vi "Rectangular Target Processing.vi"() -> ()   [LabVIEW 2011]
doc: "This VI demonstrates how to do target processing on a laptop computer. It uses the same MJPG VI as the dashboard, sets a few of the important camera properties that impact processing, and carries out the same processing steps as the RT example also included in this project."
uses:
  <vilib>/Rock Robotics/WPI/Camera/WPI_CameraImageSize.ctl
  <vilib>/Rock Robotics/WPI/Camera/WPI_CameraWhite Balance Values.ctl
  <vilib>/vision/NI_Vision_Development_Module.lvlib
panel:
  in  "Camera Settings":T2={"FPS"=30, "Compression"=30, "Image Size"=enum."320x240"}
  in  "Camera IP Address":string="192.168.0.90"
  in  "Camera Type":enum16{"206", "1011"}(ring)
  out "Target Info":T3(array[cluster])
  in  "Area Size Limit":i32=444
  in  "Particle Count Limit":i32=10
  in  "Score Limits":T4={"Rect Coverage"=76.0, "Aspect Ratio"=70.0, "X Edge Strength"=40.0, "Y Edge Strength"=60.0}
  in  "Processing":enum32{"Color", "Intensity", "Intensity Open"}(tab)
  in  "Luminance":i32=255
  in  "Saturation":i32=255
  in  "Hue":i32(knob)=65 scale=0.0..255.0
  in  "Margins":cluster{"Hue":i32, "Sat":i32, "Lum":i32}={"Hue"=9, "Sat"=40, "Lum"=19} {"Sat" scale=0.0..40.0; "Lum" scale=0.0..40.0; "Hue" scale=0.0..40.0}
  in  "Range":cluster{"Lower value":sgl, "Upper value":sgl}={"Lower value"=150.0, "Upper value"=255.0} {"Lower value" scale=0.0..255.0; "Upper value" scale=0.0..255.0}
  in  "Range":cluster{"Lower value":sgl, "Upper value":sgl}={"Lower value"=150.0, "Upper value"=255.0} {"Lower value" scale=0.0..255.0; "Upper value" scale=0.0..255.0}
  in  "Annotate":bool=TRUE
  out "Processed Image":T5(plugin-control)
  out "Original Image":T5(plugin-control)
  # "Information:\nProcessing can be based on color or light intensity.\nParticles within the image are scored by rectangle coverage, aspect ratio, and\nfor being hollow with a bold edge. A particle is considered a target if all scores\nare above the score limits you set. Particles can be annotated -- surrounded by\na rectangle and scores drawn to the left .\nTo control the number of particles being scored, use the count limit and the size\nlimit.\nBe sure to set the Camera IP before running. The distance uses the camera type\nto index lens view angle."
  # "Click in the image to select target the color for processing."
  # "Green scores are above the limit, orange are below. Inner/outer rect\nindicates all passed."
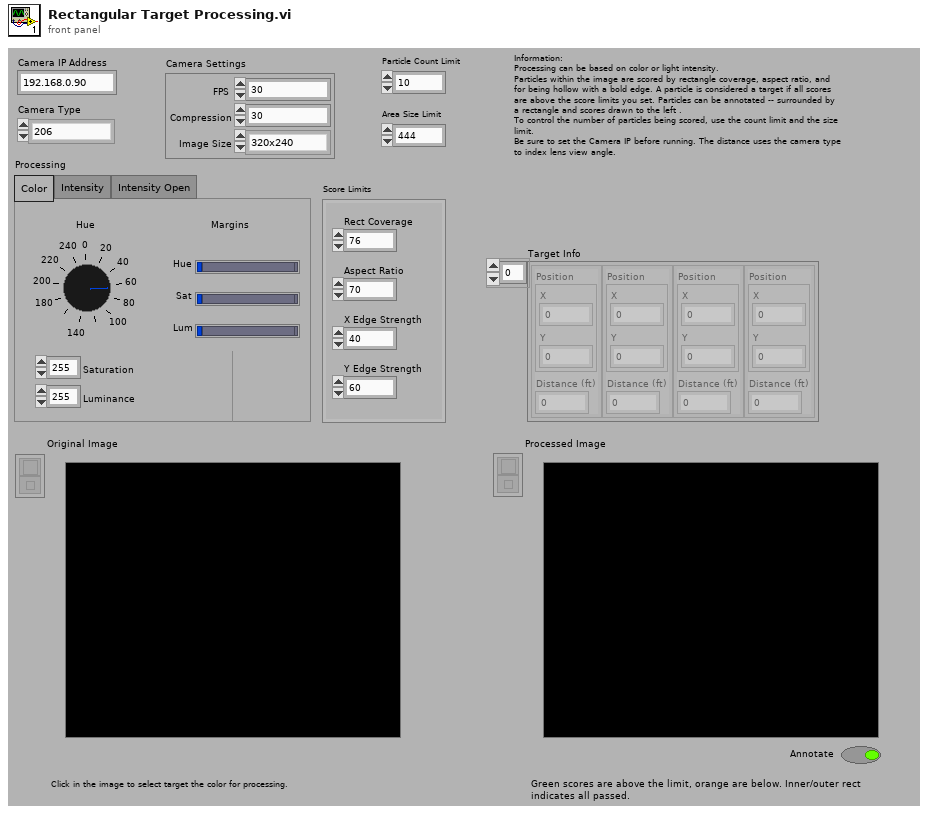
[diagram p1: front panel]
types:
  T1 = typedef "WPI_CameraImageSize.ctl" = enum16{"640x480", "320x240", "160x120"}
  T2 = cluster{"FPS":i32, "Compression":i32, "Image Size":T1}
  T3 = cluster{"Position":cluster{"X":dbl, "Y":dbl}, "Distance (ft)":dbl}[]
  T4 = cluster{"Rect Coverage":dbl, "Aspect Ratio":dbl, "X Edge Strength":dbl, "Y Edge Strength":dbl}
  T5 = typedef "IMAQ Image.ctl" = refnum<image>
  T6 = typedef "WPI_CameraWhite Balance Values.ctl" = enum16{"Auto", "Fixed indoor", "Fixed outdoor 1", "Fixed outdoor 2", "Fixed fluorescent 1", "Fixed fluorescent 2", "Hold current"}
  T7 = typedef "Image Type" = u32
  T8 = typedef "WPI_CameraDevRef.ctl" = cluster{"Camera Address":string, "CameraStatus":errorcluster, "Acquire Image Notifier":refnum<notifier>}
  T9 = enum32{"AutoM", "Close", "Dilate", "Erode", "Gradient", "Gradient out", "Gradient in", "Hit miss", "Open", "PClose", "POpen", "Thick", "Thin"}
  T10 = cluster{cluster{"Left":dbl, "Top":dbl, "Right":dbl, "Bottom":dbl}, dbl[]}[]
  T11 = cluster{"Left":dbl, "Top":dbl, "Right":dbl, "Bottom":dbl}
  T12 = cluster{"Target Center (-1 to 1)":cluster{"X":dbl, "Y":dbl}, "Distance (ft)":dbl}
  T13 = cluster{"Target Center (-1 to 1)":cluster{"X":dbl, "Y":dbl}, "Distance (ft)":dbl}[]
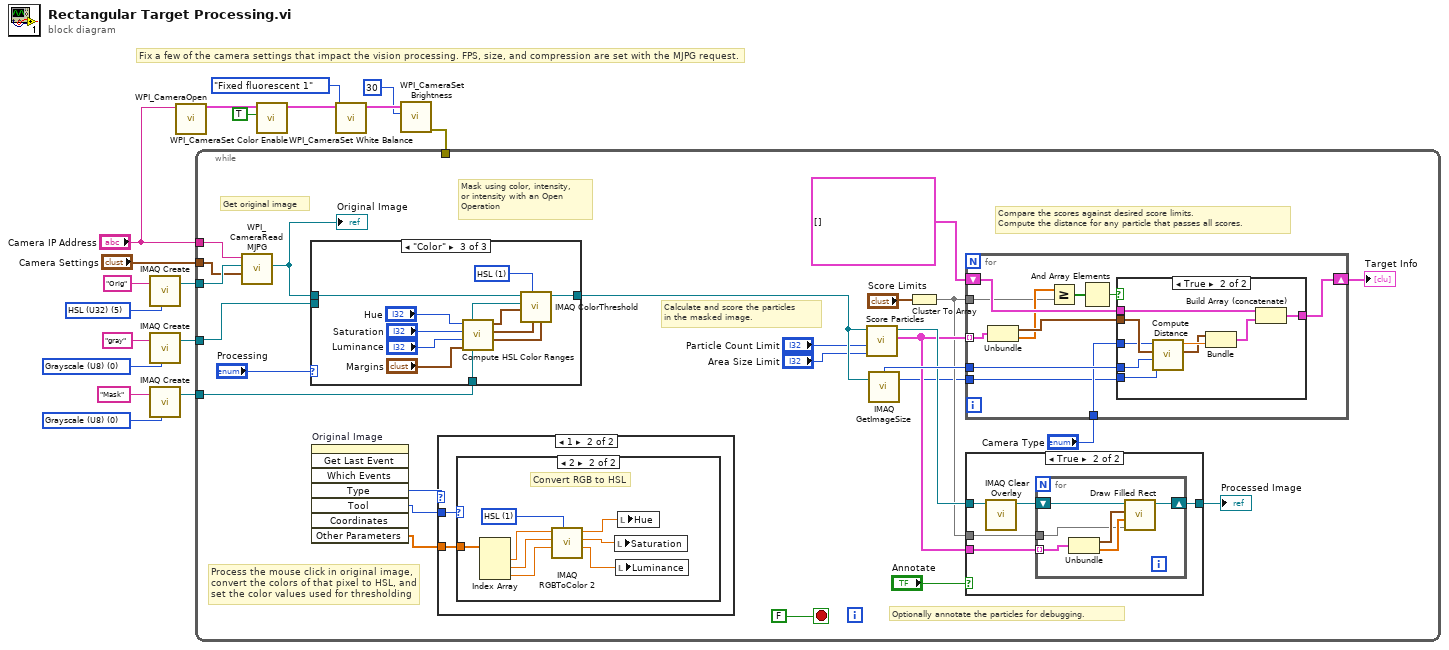
[diagram p0: block diagram]
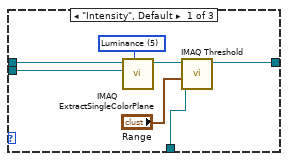
[diagram p3: hidden frame]
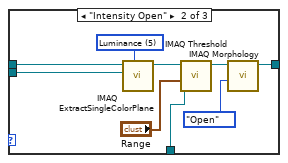
[diagram p4: hidden frame]
diagram:
  w11 = T7 0 items=["Grayscale (U8)", "Grayscale (I16)", "Grayscale (SGL)", "Complex (CSG)", "RGB (U32)", "HSL (U32)", "RGB (U64)", "Grayscale (U16)"] ("Image Type")
  w15 = T7 5 items=["Grayscale (U8)", "Grayscale (I16)", "Grayscale (SGL)", "Complex (CSG)", "RGB (U32)", "HSL (U32)", "RGB (U64)", "Grayscale (U16)"] ("Image Type")
  w18 = T7 0 items=["Grayscale (U8)", "Grayscale (I16)", "Grayscale (SGL)", "Complex (CSG)", "RGB (U32)", "HSL (U32)", "RGB (U64)", "Grayscale (U16)"] ("Image Type")
  # "Fix a few of the camera settings that impact the vision processing. FPS, size, and compression are set with the MJPG request."
  n1 = call "IMAQ Create"("Image Name"="Orig", "Image Type"=w15) -> ("New Image"=w14:T5)  [unwired: 2 in, 2 out]
  n2 = call "IMAQ Create"("Image Name"="gray", "Image Type"=w18) -> ("New Image"=w13:T5)  [unwired: 2 in, 2 out]
  n3 = call "IMAQ Create"("Image Name"="Mask", "Image Type"=w11) -> ("New Image"=w10:T5)  [unwired: 2 in, 2 out]
  n4 = call <vilib>:"WPI_CameraOpen.vi"("Camera Address"="Camera IP Address") -> ("CameraDevRef"=w8:T8)  [unwired: 9 in, 1 out]
  n5 = call <vilib>:"WPI_CameraSet Color Enable.vi"("Color Enabled"=TRUE, "CameraDevRef"=w8) -> ("CameraDevRef Out"=w6:T8)  [unwired: 8 in, 1 out]
  n6 = call <vilib>:"WPI_CameraSet White Balance.vi"("White Balance"=WPI_CameraWhite_Balance_Values."Fixed fluorescent 1", "CameraDevRef"=w6) -> ("CameraDevRef Out"=w4:T8)  [unwired: 8 in, 1 out]
  n7 = call <vilib>:"WPI_CameraSet Brightness.vi"("Brightness"=30, "CameraDevRef"=w4) -> ("error out"=w2:errorcluster)  [unwired: 8 in, 1 out]
  n8 = while {
    tunnel: w14 -> [w34]
    tunnel: w13 -> [w43]
    tunnel: w10 -> [w42]
    tunnel: "Camera IP Address" -> [w32]
    tunnel: w2 -> [_]
    tunnel: "Camera Settings" -> [w19]
    stop <- FALSE stop-if-true
    # "Optionally annotate the particles for debugging."
    # "Compare the scores against desired score limits.\nCompute the distance for any particle that passes all scores."
    # "Process the mouse click in original image,\nconvert the colors of that pixel to HSL, and\nset the color values used for thresholding"
    # "Calculate and score the particles\nin the masked image."
    # "Mask using color, intensity,\nor intensity with an Open\nOperation"
    # "Get original image"
    n9 = call <vilib>:"WPI_CameraRead MJPG.vi"("Camera Settings"=w19, "Image"=w34, "address"=w32) -> ("Image Out"=w33:T5)  [unwired: 7 in, 1 out]
    "Original Image" <- w33
    n10 = case shown="\"Color\"" "Processing" {
      tunnel: w33 -> [w62 w71 w82]
      tunnel: w43 -> [w61 w70 _]
      tunnel: w42 -> [w59 w68 w81]
      tunnel: [w57 w64 w80] -> w24
      frame "Intensity", Default {
        w56 = 5 items=["Red", "Green", "Blue", "Hue", "Saturation", "Luminance", "Value", "Intensity"] ("Color Plane")
        n11 = call "IMAQ ExtractSingleColorPlane"("Color Plane"=w56, "Image Dst"=w61, "Image Src"=w62) -> ("Image Dst Out"=w60:T5)  [unwired: 1 in, 7 out]
        n12 = call "IMAQ Threshold"("Range"="Range", "Image Dst"=w59, "Image Src"=w60) -> ("Image Dst Out"=w57:T5)  [unwired: 3 in, 5 out]
      }
      frame "Intensity Open" {
        w63 = 5 items=["Red", "Green", "Blue", "Hue", "Saturation", "Luminance", "Value", "Intensity"] ("Color Plane")
        n13 = call "IMAQ ExtractSingleColorPlane"("Color Plane"=w63, "Image Dst"=w70, "Image Src"=w71) -> ("Image Dst Out"=w69:T5)  [unwired: 1 in, 7 out]
        n14 = call "IMAQ Threshold"("Range"="Range", "Image Dst"=w68, "Image Src"=w69) -> ("Image Dst Out"=w65:T5)  [unwired: 3 in, 5 out]
        n15 = call "IMAQ Morphology"("Operation"=T9."Open", "Image Src"=w65) -> ("Image Dst Out"=w64:T5)  [unwired: 8 in, 1 out]
      }
      frame "Color" {
        w79 = u16 1 items=["RGB", "HSL", "HSV", "HSI"] ("Color Mode")
        n16 = call "Compute HSL Color Ranges.vi"("Margins"="Margins", "Luminance"="Luminance", "Saturation"="Saturation", "Hue"="Hue") -> ("Lum Range"=w76:cluster{i32, i32}, "Sat Range"=w77:cluster{i32, i32}, "Hue Range"=w78:cluster{i32, i32})  [unwired: 5 in]
        n17 = call "IMAQ ColorThreshold"("Blue or Luma or Val or Inten Range"=w76, "Green or Sat Range"=w77, "Color Mode"=w79, "Red or Hue Range"=w78, "Image Dst"=w81, "Image Src"=w82) -> ("Image Dst Out"=w80:T5)  [unwired: 4 in, 1 out]
      }
    }
    n18 = invoke on="Original Image" class="ImageControl" method="Get Last Event"() -> ("Type"=w36:i32, "Tool"=w37:i32, "Other Parameters"=w38:sgl[])  [unwired: 8 in, 5 out]
    n19 = case shown="1" w36 {
      tunnel: w37 -> [_ w105]
      tunnel: w38 -> [_ w104]
      frame 0, Default {
      }
      frame 1 {
        n20 = case shown="2" w105 {
          tunnel: w104 -> [_ w113]
          frame Default {
          }
          frame 2 {
            w112 = u16 1 items=["RGB", "HSL", "HSV", "HSI", "CIE L*a*b*", "CIE XYZ"] ("Color Mode")
            # "Convert RGB to HSL"
            n21 = Index Array(array=w113) -> (element #1=w111:sgl, element #2=w109:sgl, element #3=w107:sgl)  [unwired: 3 in]
            n22 = call "IMAQ RGBToColor 2"("Color Mode"=w112, "Blue value"=w107, "Green value"=w109, "Red value"=w111) -> ("Blue or Luma or Val or Inten or Z or b*value"=w106:dbl, "Green or Sat or Y or a* value"=w108:dbl, "Red or Hue or X or L* value"=w110:dbl)  [unwired: 4 in, 1 out]
            n23 = local write "Saturation"(w108) -> ()
            n24 = local write "Luminance"(w106) -> ()
            n25 = local write "Hue"(w110) -> ()
          }
        }
      }
    }
    n26 = call "Score Particles.vi"("Area Size Limit"="Area Size Limit", "Particle Count Limit"="Particle Count Limit", "Image Refnum in"=w24) -> ("Scored Particle Info"=w27:T10, "Image Refnum out"=w31:T5)  [unwired: 7 in]
    n27 = call "IMAQ GetImageSize"("Image"=w24) -> ("Y Resolution"=w20:i32, "X Resolution"=w35:i32)  [unwired: 3 in, 1 out]
    n28 = Cluster To Array(cluster="Score Limits") -> (array=w25:dbl[])
    n29 = for {
      shift-right: [w92] -> w39
      shift-left: T3 [] -> [w93]
      tunnel: w35 -> [w91]
      tunnel: w27 -> [w89] mode=indexing
      tunnel: w25 -> [w84]
      tunnel: "Camera Type" -> [w88]
      tunnel: w20 -> [w83]
      n30 = Unbundle(w89) -> (w90:T11, w85:dbl[])
      n31 = Greater Or Equal?(x=w85, y=w84) -> (x >= y?=w87:bool[])
      n32 = And Array Elements(Boolean array=w87) -> (logical AND=w86:bool)
      n33 = case shown="True" w86 {
        tunnel: w93 -> [w94 w103]
        tunnel: [w94 w102] -> w92
        tunnel: w90 -> [_ w98]
        tunnel: w91 -> [_ w100]
        tunnel: w88 -> [_ w97]
        tunnel: w83 -> [_ w95]
        frame False {
        }
        frame True {
          n34 = call "Compute Distance.vi"("Y Image Resolution"=w95, "X Image Resolution"=w100, "Bounding Box"=w98, "Camera Type"=w97) -> ("Target Center (-1 to 1)"=w96:cluster{"X":dbl, "Y":dbl}, "Distance (ft)"=w99:dbl)  [unwired: 6 in]
          n35 = Bundle("Target Center (-1 to 1)"=w96, "Distance (ft)"=w99) -> (w101:T12)  [unwired: 1 in]
          n36 = Build Array (concatenate)(w103, w101) -> (w102:T13)
        }
      }
    }
    "Target Info" <- w39
    n37 = case shown="True" "Annotate" {
      tunnel: w31 -> [w44 w49]
      tunnel: [w44 w48] -> w28
      tunnel: w27 -> [_ w46]
      tunnel: w25 -> [_ w45]
      frame False {
      }
      frame True {
        n38 = call "IMAQ Clear Overlay"("Image"=w49) -> ("Image Out"=w47:T5)  [unwired: 2 in, 8 out]
        n39 = for {
          shift-right: [w54] -> w48
          shift-left: w47 -> [w55]
          tunnel: w46 -> [w51] mode=indexing
          tunnel: w45 -> [w50]
          n40 = Unbundle(w51) -> (w52:T11, w53:dbl[])
          n41 = call "Draw Filled Rect.vi"("Limits"=w50, "Scores"=w53, "Bounding Box"=w52, "image in"=w55) -> ("image out"=w54:T5)  [unwired: 7 in]
        }
      }
    }
    "Processed Image" <- w28
  }
